vi "Get Project Paths.vi"() -> (1 "PlatformIO lib path":path, 2 "Firmware path":path, 3 "Repo Base":path)   [LabVIEW 2019, in "LINXx.lvlib"]
doc: "Dev helper to locate key paths in the project"
uses:
  LINXx.lvlib
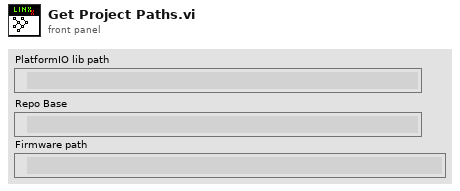
[diagram p1: front panel]
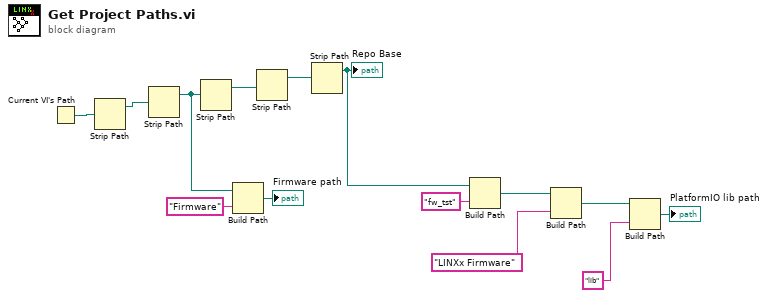
[diagram p0: block diagram]
diagram:
  n1 = Current VI's Path() -> (path=w14:path)
  n2 = Strip Path(path=w14) -> (stripped path=w13:path)  [unwired: 1 out]
  n3 = Strip Path(path=w13) -> (stripped path=w10:path)  [unwired: 1 out]
  n4 = Strip Path(path=w10) -> (stripped path=w12:path)  [unwired: 1 out]
  n5 = Build Path(base path=w10, name or relative path="Firmware") -> (appended path=→"Firmware path":path)
  n6 = Strip Path(path=w12) -> (stripped path=w11:path)  [unwired: 1 out]
  n7 = Strip Path(path=w11) -> (stripped path=w2:path)  [unwired: 1 out]
  "Repo Base" <- w2
  n8 = Build Path(base path=w2, name or relative path="fw_tst") -> (appended path=w6:path)
  n9 = Build Path(base path=w6, name or relative path="LINXx Firmware") -> (appended path=w5:path)
  n10 = Build Path(base path=w5, name or relative path="lib") -> (appended path=→"PlatformIO lib path":path)
